vi "Temperature.vi"(7 "Address":u16, 8 "Error In":errorcluster, 11 "VISA Resource in":refnum<visa-resource-name>) -> (0 "Error Out":errorcluster, 2 "Temperature":dbl[unit]=273.15, 3 "VISA Resource out":refnum<visa-resource-name>)   [LabVIEW 2014, in "KIT QV.lvlib"]
doc: "Averaged temperature of all marked detectors."
uses:
  KIT QV.lvlib
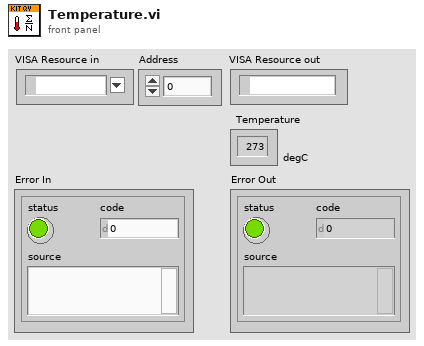
[diagram p1: front panel]
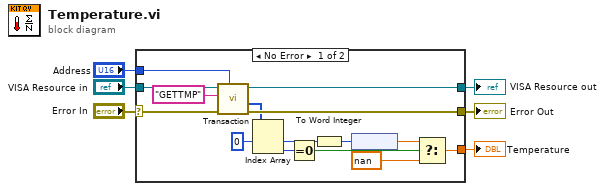
[diagram p0: block diagram]
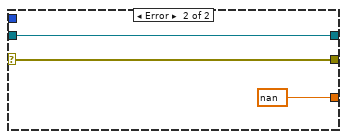
[diagram p2: hidden frame]
diagram:
  n1 = case shown="No Error" "Error In" {
    selector: "Error In" -> [w20 w23]
    tunnel: [w17 w24] -> w6
    tunnel: [w16 w23] -> w5
    tunnel: "VISA Resource in" -> [w21 w24]
    tunnel: "Address" -> [w18 _]
    tunnel: [w8 dbl[unit] nan ("f")] -> w1
    frame No Error {
      n2 = call "Transaction.vi"("Address"=w18, "error in (no error)"=w20, "Command"="GETTMP" ("Reset Command"), "VISA Resource in"=w21) -> ("error out"=w16:errorcluster, "Parameter out"=w15:u8[], "VISA Resource out"=w17:refnum<visa-resource-name>)  [unwired: 5 in]
      n3 = Index Array(array=w15, index #1=0 ("index")) -> (element #1=w13:u8, element #2=w12:u8)  [unwired: 1 in]
      n4 = Equal To 0?(x=w12) -> (x = 0?=w10:bool)
      n5 = To Word Integer(number=w13) -> (16bit integer=w7:i16)
      n6 = node(w7) -> (w11:dbl[unit])
      n7 = Select(t=w11, s=w10, f=dbl[unit] nan) -> (s? t:f=w8:dbl[unit])
    }
    frame Error {
    }
  }
  "Error Out" <- w5
  "VISA Resource out" <- w6
  "Temperature" <- w1
